vi "Do.vi"(8 "error in":errorcluster, 10 "Actor in":refnum<class "Actor.lvclass">, 11 "Speaker MSG":refnum<class "Speaker MSG.lvclass">) -> (0 "error out":errorcluster, 2 "Actor out":refnum<class "Actor.lvclass">)   [LabVIEW 2014, in "Controller.lvlib" / "Speaker MSG.lvclass"]
doc: "Forward a message to the PAS object to toggle the speaker position."
uses:
  Speaker MSG.lvclass
  <vilib>/ActorFramework/Actor/Actor.lvclass
  Controller.lvclass
  Controls/eMap.ctl
  <vilib>/ActorFramework/Message Enqueuer/Message Enqueuer.lvclass
  Speaker MSG.lvclass/Speaker MSG.ctl
  Controller.lvclass/Controller.ctl
  SuperActor/SuperActor.lvclass/SuperActor.ctl
  Instr Actor/Messages/Change Speaker State/Change Speaker Switch MSG.lvclass
  Update Switch State MSG/Update Switch MSG.lvclass/Update Switch MSG.ctl
  <vilib>/ActorFramework/Message Enqueuer/Message Enqueuer.lvclass/Message Enqueuer.ctl
  Update Switch State MSG/Write SwitchState.vi
  Accessors/Read Enqueuer Map.vi
  SuperActor/Read Log Session.vi
  <vilib>/ActorFramework/Message Priority Queue/Priority Enqueue.vi
  <userlib>/_Session Fwk/Session - Root.lvclass
  reusable/Session APIs/Session Log/System Log.lvclass
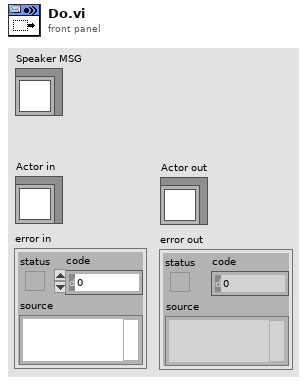
[diagram p1: front panel]
types:
  T1 = typedef "Controller.lvlib/Controller.lvclass/eMap.ctl" = cluster{"Enqueuer":refnum<class "Message Enqueuer.lvclass">, "Active":bool}
  T2 = typedef "Session - Root.lvclass/Session Handle.ctl" = refnum<data-value>
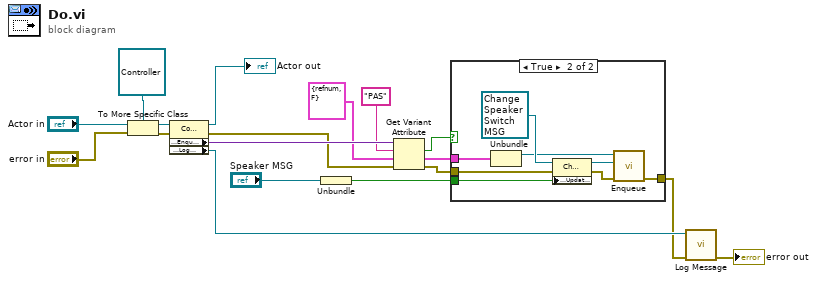
[diagram p0: block diagram]
diagram:
  n1 = To More Specific Class(target class=refnum<class "Controller.lvclass"> refnum ("Controller:Controller"), reference="Actor in", error in="error in") -> (specific class reference=w16:refnum<class "Controller.lvclass">, error out=w6:errorcluster)
  n2 = property class="Controller"(reference=w16, error in=w6) -> (reference out=→"Actor out":refnum<class "Controller.lvclass">, error out=w10:errorcluster, "Accessors:Enqueuer Map"=w13:variant, "Accessors:Log Session"=w3:T2)
  n3 = Unbundle("Speaker MSG") -> (w14:bool)
  n4 = Get Variant Attribute(Variant=w13, name="PAS", default value (empty Variant)=T1 {"Enqueuer"=refnum, "Active"=FALSE} ("eMap"), error in=w10) -> (found=w9:bool, value=w8:T1, error out=w5:errorcluster)  [unwired: 1 out]
  n5 = case shown="True" w9 {
    tunnel: w14 -> [_ w26]
    tunnel: w8 -> [_ w24]
    tunnel: w5 -> [w19 w22]
    tunnel: [w19 w20] -> w2
    frame False {
    }
    frame True {
      n6 = Unbundle(w24) -> ("Enqueuer"=w23:refnum<class "Message Enqueuer.lvclass">)  [unwired: 1 out]
      n7 = property class="Change Speaker MSG"(reference=refnum<class "Change Speaker Switch MSG.lvclass"> refnum ("ePAS Library.lvlib:Change Speaker MSG"), error in=w22, "Accessors:UpdateSw"=w26) -> (reference out=w25:refnum<class "Change Speaker Switch MSG.lvclass">, error out=w21:errorcluster)
      n8 = call <vilib>:"Enqueue.vi"("error in (no error)"=w21, "Message"=w25, "Message Enqueuer in"=w23) -> ("error out"=w20:errorcluster)  [unwired: 7 in, 1 out]
    }
  }
  n9 = call "Log Message.vi"("error in"=w2, "session in"=w3) -> ("error out"=→"error out":errorcluster)  [unwired: 8 in, 1 out]
